vi "GetWAFactor.vi"(8 "error in (no error)":errorcluster, 11 "Laser Diode Controller in":refnum<class "KLD101.lvclass">) -> (0 "error out":errorcluster, 2 "waFactor":dbl, 3 "Laser Diode Controller out":refnum<class "KLD101.lvclass">)   [LabVIEW 2016, in "Laser Diode Controller.lvlib" / "KLD101.lvclass"]
uses:
  KLD101.lvclass
  KLD101.lvclass/KLD101.ctl
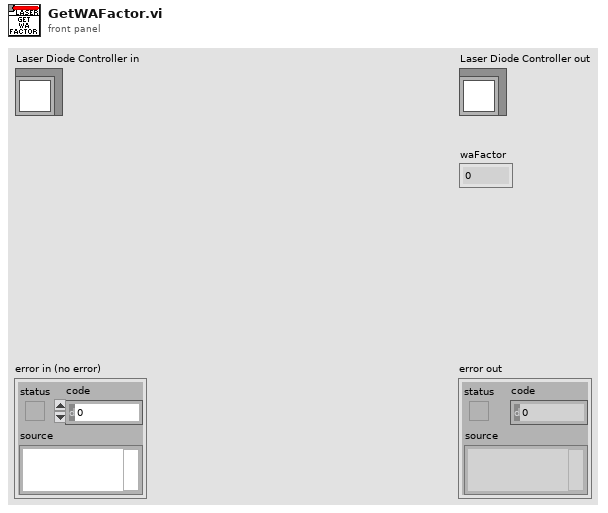
[diagram p1: front panel]
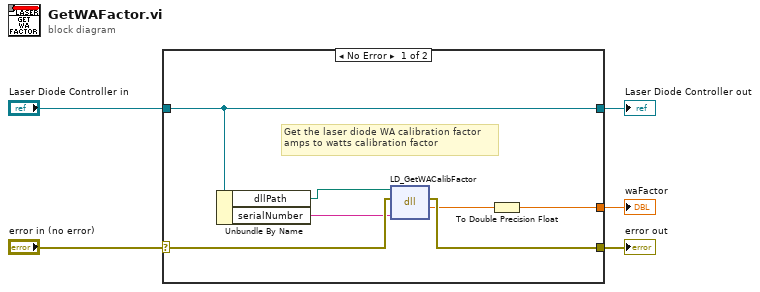
[diagram p0: block diagram]
diagram:
  n1 = case shown="No Error" "error in (no error)" {
    selector: "error in (no error)" -> [w11 w14]
    tunnel: [w10 w14] -> w4
    tunnel: [w12 w13] -> w2
    tunnel: "Laser Diode Controller in" -> [w12 w13]
    tunnel: [w7 _] -> w1
    frame No Error {
      # "Get the laser diode WA calibration factor\namps to watts calibration factor"
      n2 = Unbundle By Name(w12) -> ("dllPath"=w6:path, "serialNumber"=w8:string)
      n3 = dll-call lib="C:/IDEXX Software/Collimation/data/Thorlabs.MotionControl.KCube.LaserDiode.dll" fn="LD_GetWACalibFactor"(path in=w6, error in=w11, "serialNumber"=w8) -> (error out=w10:errorcluster, "current"=w9:sgl)  [unwired: 2 in, 1 out]
      n4 = To Double Precision Float(number=w9) -> (double precision float=w7:dbl)
    }
    frame Error {
    }
  }
  "error out" <- w4
  "Laser Diode Controller out" <- w2
  "waFactor" <- w1
